vi "Hardware Status Logic (SubVI).vi"(8 "Error":bool, 11 "error in (no error)":errorcluster) -> (0 "Hardware status":bool, 3 "error out":errorcluster)   [LabVIEW 2014]
uses:
  <vilib>/rvi/eio/common/nirviEmuTemplateMethod_errors.vi
  <vilib>/eio/EIOMethodNode/EIOMethodNode.xnode
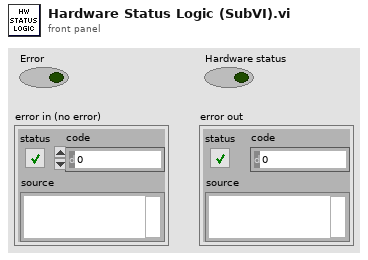
[diagram p1: front panel]
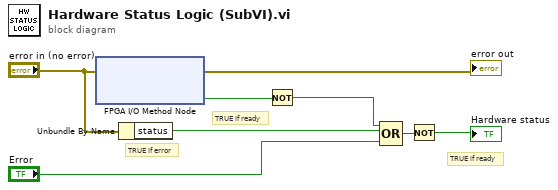
[diagram p0: block diagram]
diagram:
  # "TRUE if ready"
  # "TRUE if ready"
  # "TRUE if error"
  n1 = xnode "FPGA I/O Method Node"("error in"="error in (no error)") -> ("error out"=→"error out":errorcluster, "Ready"=w6:bool)  [unwired: 1 in, 1 out]
  n2 = Unbundle By Name("error in (no error)") -> ("status"=w7:bool)
  n3 = Not(x=w6) -> (.not. x?=w5:bool)
  n4 = Compound Arithmetic op=OR(w5, w7, "Error") -> (w2:bool)
  n5 = Not(x=w2) -> (.not. x?=→"Hardware status":bool)
